vi "AutoForwardOrBack.vi"(10 "Case":string, 11 "Drive Speed":dbl) -> ()   [LabVIEW 2016]
uses:
  <vilib>/Rock Robotics/WPI/Utilities/WPI_GetSetVariantRefNum.vi
  <vilib>/Rock Robotics/WPI/RobotDrive/WPI_RobotDriveMecanumDrive_Cartesian.vi
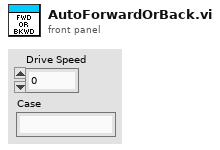
[diagram p1: front panel]
types:
  T1 = typedef "WPI_RobotDriveDevRef.ctl" = cluster{"DevStatus":errorcluster, "Motors[]":T2[], "Square Inputs":bool, "Max Output":dbl}
  T2 = typedef "WPI_MotorControlDeviceRef.ctl" = cluster{"DeviceStatus":errorcluster, "Type":T3, "PWM":cluster{"PWM Channel":T4, "DeadBand":T5}, "CAN":cluster{"Device Number":u8, "SetOutput VI Ref":variant, "GetOutput VI Ref":variant, "Enable VI Ref":variant, "Disable VI Ref":variant, "Data":variant}, "Invert":bool}
  T3 = typedef "WPI_MotorControlType.ctl" = enum16{"PWM", "CAN"}
  T4 = typedef "FPGA_DIOPWMChannel.ctl" = enum8{"PWM 0", "PWM 1", "PWM 2", "PWM 3", "PWM 4", "PWM 5", "PWM 6", "PWM 7", "PWM 8", "PWM 9", "PWM MXP 0", "PWM MXP 1", "PWM MXP 2", "PWM MXP 3", "PWM MXP 4", "PWM MXP 5", "PWM MXP 6", "PWM MXP 7", "PWM MXP 8", "PWM MXP 9", "Invalid"}
  T5 = typedef "WPI_PWMDeadband.ctl" = cluster{"Name":string, "maxPositivePwm":i32, "minPositivePwm":i32, "centerPwm":i32, "maxNegativePwm":i32, "minNegativePwm":i32, "angularRange":u16}
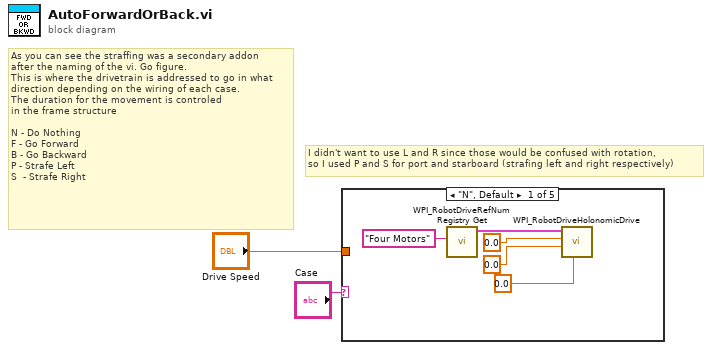
[diagram p0: block diagram]
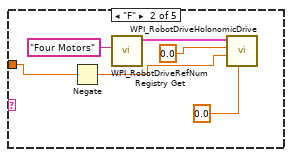
[diagram p2: hidden frame]
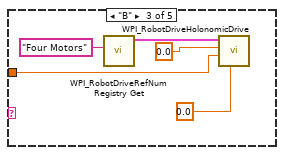
[diagram p3: hidden frame]
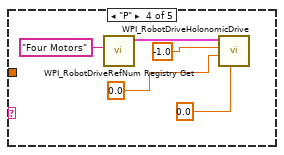
[diagram p4: hidden frame]
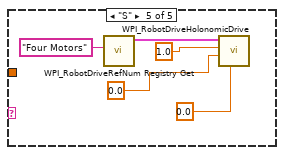
[diagram p5: hidden frame]
diagram:
  # "As you can see the straffing was a secondary addon\nafter the naming of the vi. Go figure.\nThis is where the drivetrain is addressed to go in what\ndirection depending on the wiring of each case.\nThe duration for the movement is controled\nin the frame structure  \n\nN - Do Nothing\nF - Go Forward\nB - Go Backward\nP - Strafe Left\nS  - Strafe Right"
  # "I didn't want to use L and R since those would be confused with rotation,\nso I used P and S for port and starboard (strafing left and right respectively)"
  n1 = case shown="\"N\", Default" "Case" {
    tunnel: "Drive Speed" -> [_ w9 w16 _ _]
    frame "N", Default {
      n2 = call <vilib>:"WPI_RobotDriveRefNum Registry Get.vi"("refnum name"="Four Motors") -> ("RobotDriveDevRef"=w7:T1)  [unwired: 9 in, 1 out]
      n3 = call-poly <vilib>:"WPI_RobotDriveHolonomicDrive.vi"("Rotation"=0.0, "Y"=0.0, "X"=0.0, "RobotDriveDevRef"=w7) -> ()  [unwired: 5 in, 3 out]
    }
    frame "F" {
      n4 = Negate(x=w9) -> (-x=w8:dbl)
      n5 = call <vilib>:"WPI_RobotDriveRefNum Registry Get.vi"("refnum name"="Four Motors") -> ("RobotDriveDevRef"=w13:T1)  [unwired: 9 in, 1 out]
      n6 = call-poly <vilib>:"WPI_RobotDriveHolonomicDrive.vi"("Rotation"=0.0 ("X"), "Y"=w8, "X"=0.0 ("Y"), "RobotDriveDevRef"=w13) -> ()  [unwired: 5 in, 3 out]
    }
    frame "B" {
      n7 = call <vilib>:"WPI_RobotDriveRefNum Registry Get.vi"("refnum name"="Four Motors") -> ("RobotDriveDevRef"=w18:T1)  [unwired: 9 in, 1 out]
      n8 = call-poly <vilib>:"WPI_RobotDriveHolonomicDrive.vi"("Rotation"=0.0 ("X"), "Y"=w16, "X"=0.0 ("Y"), "RobotDriveDevRef"=w18) -> ()  [unwired: 5 in, 3 out]
    }
    frame "P" {
      n9 = call <vilib>:"WPI_RobotDriveRefNum Registry Get.vi"("refnum name"="Four Motors") -> ("RobotDriveDevRef"=w23:T1)  [unwired: 9 in, 1 out]
      n10 = call-poly <vilib>:"WPI_RobotDriveHolonomicDrive.vi"("Rotation"=0.0 ("X"), "Y"=0.0, "X"=-1.0 ("Y"), "RobotDriveDevRef"=w23) -> ()  [unwired: 5 in, 3 out]
    }
    frame "S" {
      n11 = call <vilib>:"WPI_RobotDriveRefNum Registry Get.vi"("refnum name"="Four Motors") -> ("RobotDriveDevRef"=w28:T1)  [unwired: 9 in, 1 out]
      n12 = call-poly <vilib>:"WPI_RobotDriveHolonomicDrive.vi"("Rotation"=0.0 ("X"), "Y"=0.0, "X"=1.0 ("Y"), "RobotDriveDevRef"=w28) -> ()  [unwired: 5 in, 3 out]
    }
  }
